vi "生成数据合成.vi"(1 "datas":string[](array[string]), 2 "fields":string[](array[string])) -> (0 "fields-datas":string)   [LabVIEW 2020]
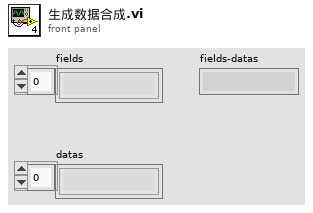
[diagram p1: front panel]
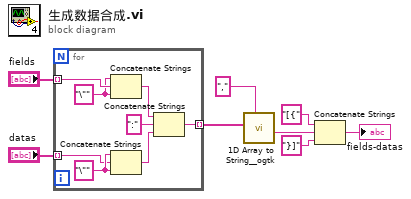
[diagram p0: block diagram]
diagram:
  n1 = for {
    tunnel: "fields" -> [w16] mode=indexing
    tunnel: "datas" -> [w11] mode=indexing
    tunnel: [w9] -> w3 mode=indexing
    w12 = "\""
    w15 = "\""
    n2 = Concatenate Strings(w15, w16, w15) -> (w14:string)
    n3 = Concatenate Strings(w12, w11, w12) -> (w10:string)
    n4 = Concatenate Strings(w14, ":", w10) -> (w9:string)
  }
  n5 = call <userlib>:"1D Array to String__ogtk.vi"("delimiter (Tab)"=",", "Array of Strings"=w3) -> ("delimited string"=w5:string)  [unwired: 9 in]
  n6 = Concatenate Strings("[{", w5, "}]") -> (→"fields-datas":string)
